vi "testSplashScreen.vi"() -> ()   [LabVIEW 2014]
panel:
  in  "stop":bool
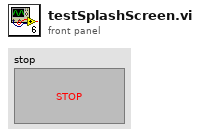
[diagram p1: front panel]
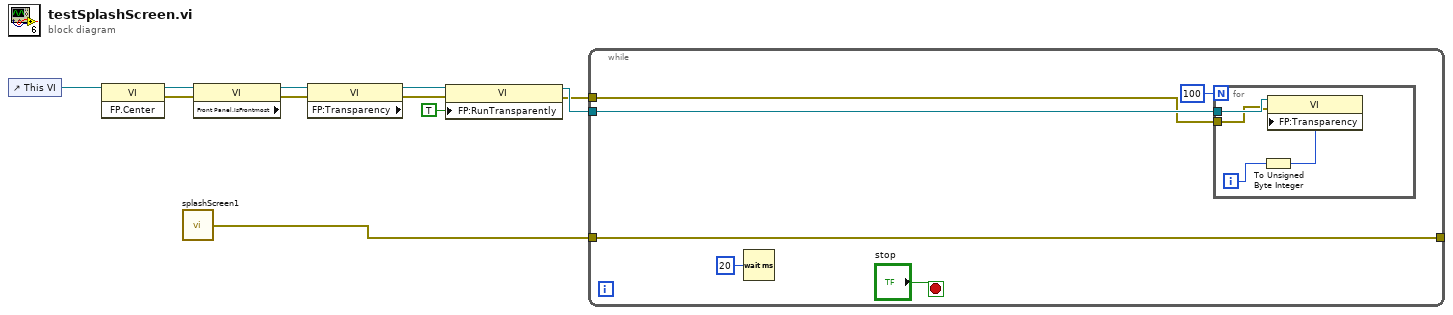
[diagram p0: block diagram]
diagram:
  n1 = control-ref of="This VI"() -> (w10:refnum<vi>)
  n2 = invoke class="VI" method="FP.Center"(reference=w10) -> (reference out=w9:refnum<vi>, error out=w8:errorcluster)  [unwired: 2 in, 1 out]
  n3 = call "splashScreen1.vi"() -> ("error out"=w11:errorcluster)  [unwired: 1 in]
  n4 = property class="VI" props=["Front Panel.IsFrontmost"](reference=w9, error in=w8) -> (reference out=w7:refnum<vi>, error out=w6:errorcluster)  [unwired: 1 out]
  n5 = property class="VI" props=["FP:Transparency"](reference=w7, error in=w6) -> (reference out=w4:refnum<vi>, error out=w3:errorcluster)  [unwired: 1 out]
  n6 = property class="VI"(reference=w4, error in=w3, "FP:RunTransparently"=TRUE ("Front Panel Window:Run VI Transparently")) -> (reference out=w2:refnum<vi>, error out=w1:errorcluster)
  n7 = while {
    tunnel: w11 -> [w12]
    tunnel: w2 -> [w14]
    tunnel: w1 -> [w13]
    tunnel: [w12] -> _
    stop <- "stop" stop-if-true
    n8 = Wait (ms)(milliseconds to wait=u32 20) -> ()  [unwired: 1 out]
    n9 = for {
      N: 100 -> [_]
      tunnel: w14 -> [w21]
      tunnel: w13 -> [w18]
      i -> [w20]
      n10 = To Unsigned Byte Integer(number=w20) -> (unsigned 8bit integer=w19:u8)
      n11 = property class="VI"(reference=w21, error in=w18, "FP:Transparency"=w19) -> ()  [unwired: 2 out]
    }
  }
